vi "AudioTest.Config, Deploy Config Files.vi"(8 "error in (no error)":errorcluster, 9 "SkipIfExists(F)/Overwrite(T)":bool, 11 "Config Folder":path=path "c:/MTE/Audio Test/Config") -> (0 "error out":errorcluster)   [LabVIEW 2018]
uses:
  <vilib>/KATE/Files/File Utils.lvlib
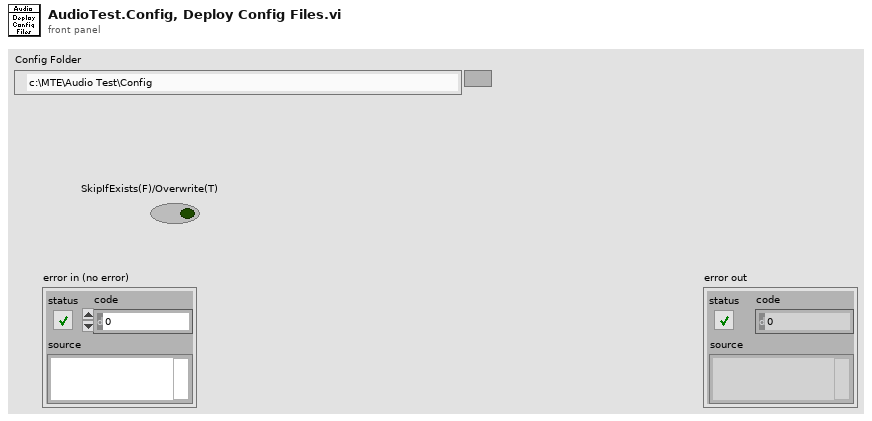
[diagram p1: front panel]
types:
  T1 = enum32{"invalid app kind", "Development System", "Run Time System", "Student Edition", "Embedded LabVIEW", "Evaluation", "Custom"}
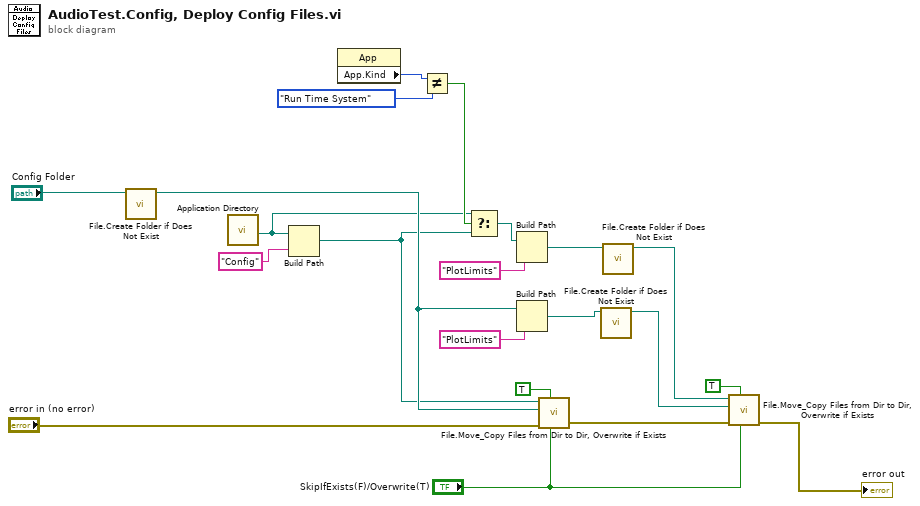
[diagram p0: block diagram]
diagram:
  n1 = call <vilib>:"File.Create Folder if Does Not Exist.vi"("Path"="Config Folder") -> ("Dup Path"=w14:path)  [unwired: 8 in, 2 out]
  n2 = call <vilib>:"Application Directory.vi"() -> ("Application Directory"=w8:path)
  n3 = Build Path(base path=w8, name or relative path="Config") -> (appended path=w7:path)
  n4 = property class="App"() -> ("App.Kind"=w11:T1)  [unwired: 2 in, 2 out]
  n5 = Not Equal?(x=w11, y=T1."Run Time System") -> (x != y?=w9:bool)
  n6 = Select(t=w8, s=w9, f=w7) -> (s? t:f=w6:path)
  n7 = Build Path(base path=w6, name or relative path="PlotLimits") -> (appended path=w5:path)
  n8 = Build Path(base path=w14, name or relative path="PlotLimits") -> (appended path=w3:path)
  n9 = call "File.Move_Copy Files from Dir to Dir, Overwrite if Exists.vi"("SkipIfExists(F)/Overwrite(T)"="SkipIfExists(F)/Overwrite(T)", "Move(F)/Copy(T)"=TRUE, "error in"="error in (no error)", "Dest Dir"=w14, "Source Dir"=w7) -> ("error out"=w13:errorcluster)  [unwired: 5 in, 1 out]
  n10 = call <vilib>:"File.Create Folder if Does Not Exist.vi"("Path"=w3) -> ("Dup Path"=w4:path)  [unwired: 8 in, 2 out]
  n11 = call <vilib>:"File.Create Folder if Does Not Exist.vi"("Path"=w5) -> ("Dup Path"=w2:path)  [unwired: 8 in, 2 out]
  n12 = call "File.Move_Copy Files from Dir to Dir, Overwrite if Exists.vi"("SkipIfExists(F)/Overwrite(T)"="SkipIfExists(F)/Overwrite(T)", "Move(F)/Copy(T)"=TRUE, "error in"=w13, "Dest Dir"=w4, "Source Dir"=w2) -> ("error out"=→"error out":errorcluster)  [unwired: 5 in, 1 out]
